vi "setMux.vi"(8 "error in (no error)":errorcluster, 10 "MUX Settings":T2, 11 "MUX Signals":T1) -> (0 "error out":errorcluster)   [LabVIEW 2015]
uses:
  Typedefs/MUX Settings.ctl
  Typedefs/Digital Signal Level.ctl
  Typedefs/MUX Signals.ctl
  Typedefs/ILCBTTypedefs.lvlib
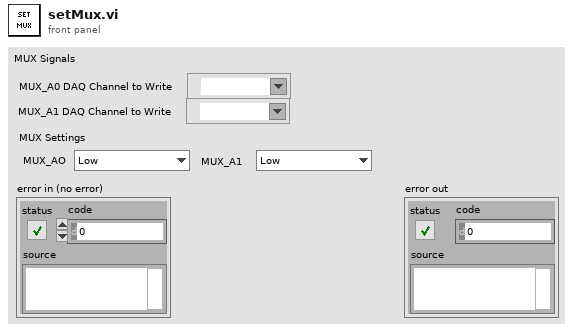
[diagram p1: front panel]
types:
  T1 = typedef "ILCBTTypedefs.lvlib/MUX Signals.ctl" = cluster{"MUX_A0 DAQ Channel to Write":refnum<k21>, "MUX_A1 DAQ Channel to Write":refnum<k21>}
  T2 = typedef "ILCBTTypedefs.lvlib/MUX Settings.ctl" = cluster{"MUX_AO":T3, "MUX_A1":T3}
  T3 = typedef "ILCBTTypedefs.lvlib/Digital Signal Level.ctl" = enum16{"Low", "High"}
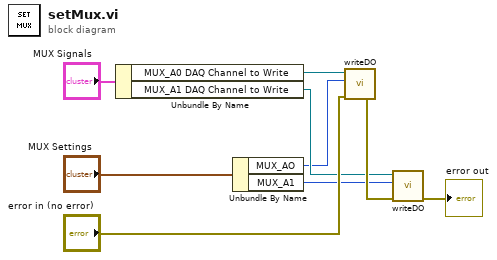
[diagram p0: block diagram]
diagram:
  n1 = Unbundle By Name("MUX Signals") -> ("MUX_A0 DAQ Channel to Write"=w4:refnum<k21>, "MUX_A1 DAQ Channel to Write"=w3:refnum<k21>)
  n2 = Unbundle By Name("MUX Settings") -> ("MUX_AO"=w2:T3, "MUX_A1"=w1:T3)
  n3 = call "writeDO.vi"("error in"="error in (no error)", "Digital Signal Level"=w2, "DAQmx Global Channel"=w4) -> ("error out"=w6:errorcluster)  [unwired: 8 in]
  n4 = call "writeDO.vi"("error in"=w6, "Digital Signal Level"=w1, "DAQmx Global Channel"=w3) -> ("error out"=→"error out":errorcluster)  [unwired: 8 in]
